vi "Data File Create.vi"(8 "error in (no error)":errorcluster, 11 "Acq and Logging Props":T1) -> (0 "error out":errorcluster, 3 "TDMS File Reference":refnum<k34>)   [LabVIEW 2013]
uses:
  Global - Configuration.vi
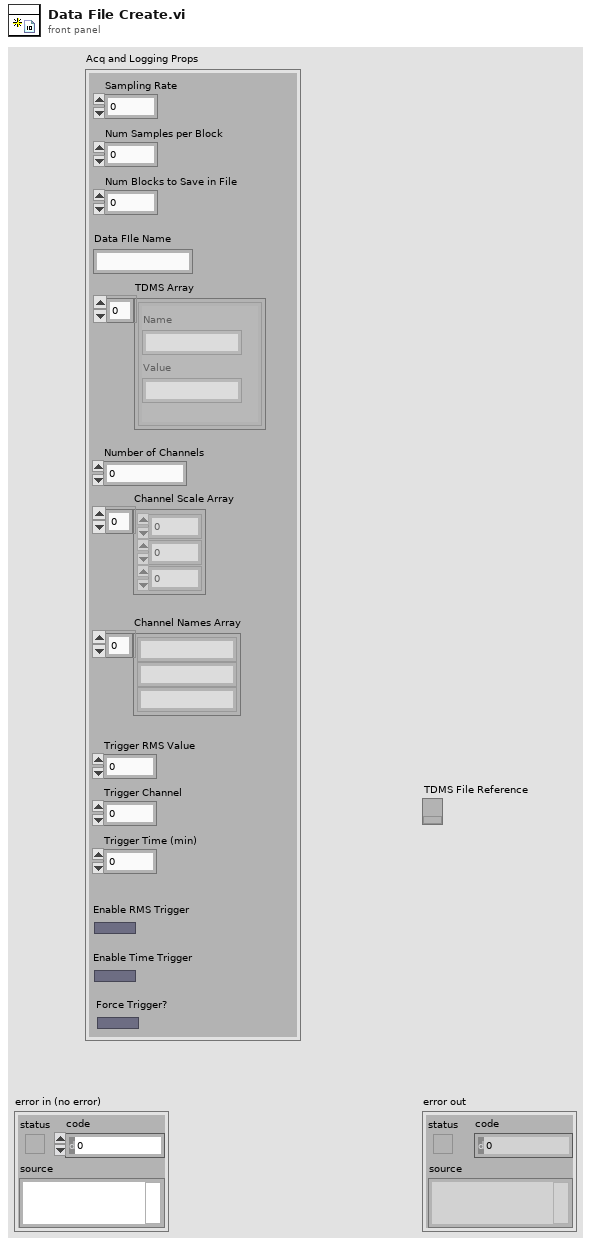
[diagram p1: front panel]
types:
  T1 = cluster{"Sampling Rate":dbl, "Num Samples per Block":i32, "Num Blocks to Save in File":i32, "Data FIle Name":string, "TDMS Array":cluster{"Name":string, "Value":string}[], "Number of Channels":i32, "Channel Scale Array":dbl[], "Channel Names Array":string[], "Trigger RMS Value":dbl, "Trigger Channel":i32, "Trigger Time (min)":i32, "Enable RMS Trigger":bool, "Enable Time Trigger":bool, "Force Trigger?":bool}
  T2 = enum16{"open", "open or create", "create or replace", "create", "open (read-only)"}
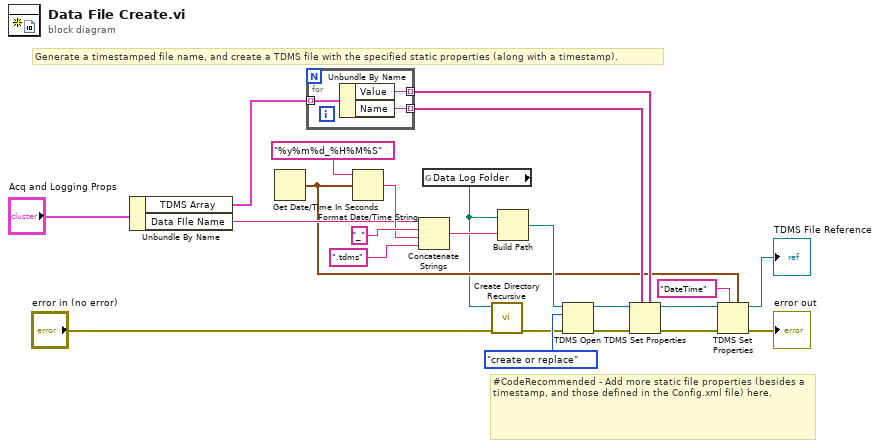
[diagram p0: block diagram]
diagram:
  # "Generate a timestamped file name, and create a TDMS file with the specified static properties (along with a timestamp)."
  # "#CodeRecommended - Add more static file properties (besides a timestamp, and those defined in the Config.xml file) here."
  n1 = Unbundle By Name("Acq and Logging Props") -> ("TDMS Array"=w13:cluster{"Name":string, "Value":string}[], "Data FIle Name"=w19:string)
  n2 = Get Date/Time In Seconds() -> (seconds since 1Jan1904=w9:timestamp)
  n3 = for {
    tunnel: w13 -> [w26] mode=indexing
    tunnel: [w25] -> w12 mode=indexing
    tunnel: [w24] -> w11 mode=indexing
    n4 = Unbundle By Name(w26) -> ("Value"=w24:string, "Name"=w25:string)
  }
  n5 = Format Date/Time String(time format string (%c)="%y%m%d_%H%M%S", seconds (now)=w9) -> (date/time string=w22:string)  [unwired: 1 out]
  n6 = Concatenate Strings(w19, "_" ("string"), w22, ".tdms" ("string")) -> (w18:string)
  n7 = global read "Global - Configuration.vi" "Data Log Folder"() -> (w2:path)
  n8 = call <vilib>:"Create Directory Recursive.vi"("error in (no error)"="error in (no error)", "directory"=w2) -> ("error out"=w4:errorcluster)  [unwired: 3 in, 2 out]
  n9 = Build Path(base path=w2, name or relative path=w18) -> (appended path=w16:path)
  n10 = TDMS Open(8:w4, 10:T2."create or replace" ("operation (0:open)"), 11:w16) -> (0:w15:errorcluster, 3:w14:refnum<k34>)  [unwired: 4 in]
  n11 = TDMS Set Properties(5:w11, 7:w12, 8:w15, 11:w14) -> (0:w10:errorcluster, 3:w6:refnum<k34>)  [unwired: 2 in, 2 out]
  n12 = TDMS Set Properties(5:w9, 7:"DateTime" ("property names"), 8:w10, 11:w6) -> (0:→"error out":errorcluster, 3:→"TDMS File Reference":refnum<k34>)  [unwired: 2 in, 2 out]
